vi "sftp.vi"() -> ()   [LabVIEW 2013]
doc: "Illustrate how to read a file using SFTP."
uses:
  libssh2/libssh2_init_default.vi
  libssh2/libssh2_session_handshake_tcp.vi
  libssh2/libssh2.lvlib
panel:
  out "total bytes read":i32
  in  "file":string="/"
  out "file content":string
  out "error out":errorcluster
  in  "password":string
  in  "username":string
  in  "hostname":string
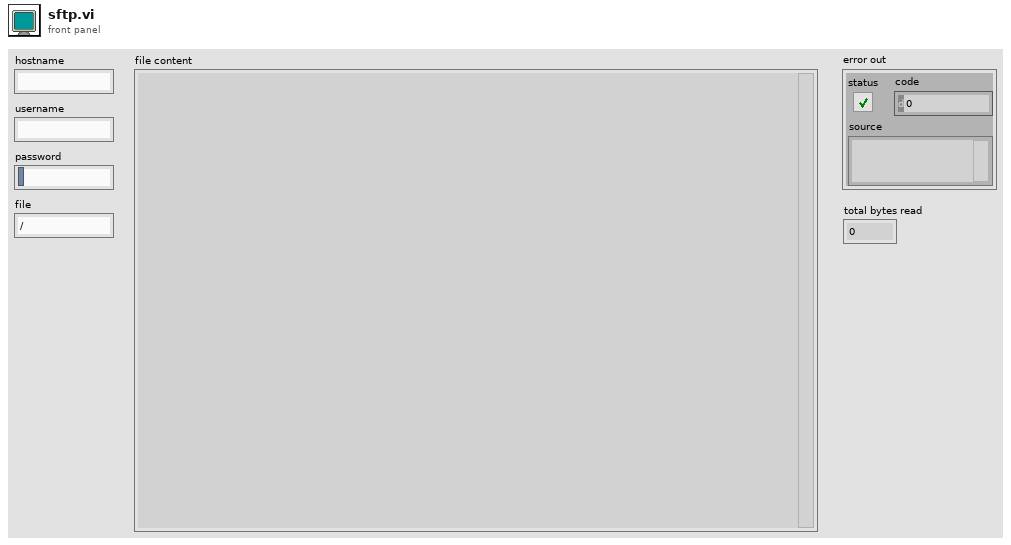
[diagram p1: front panel]
types:
  T1 = typedef "libssh2.lvlib/Session Refnum.ctl" = refnum<k1>
  T2 = typedef "libssh2.lvlib/SFTP Refnum.ctl" = refnum<k1>
  T3 = typedef "libssh2.lvlib/SFTP Handle Refnum.ctl" = refnum<k1>
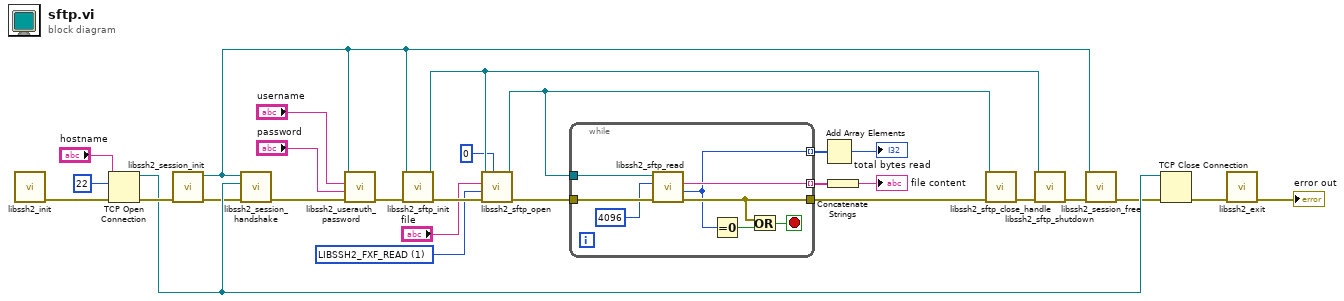
[diagram p0: block diagram]
diagram:
  w5 = u32 1 items=["LIBSSH2_FXF_READ"=1, "LIBSSH2_FXF_WRITE"=2, "LIBSSH2_FXF_APPEND"=4, "LIBSSH2_FXF_CREAT"=8, "LIBSSH2_FXF_TRUNC"=16, "LIBSSH2_FXF_EXCL"=32] ("flags")
  n1 = call-poly "libssh2_init.vi"() -> ("error out"=w27:errorcluster)  [unwired: 11 in]
  n2 = TCP Open Connection(address="hostname", remote port or service name=u16 22, error in (no error)=w27) -> (connection ID=w25:refnum<k5>, error out=w26:errorcluster)  [unwired: 2 in]
  n3 = call "libssh2_session_init.vi"("error in (no error)"=w26) -> ("error out"=w24:errorcluster, "session"=w17:T1)  [unwired: 9 in]
  n4 = call-poly "libssh2_session_handshake.vi"("error in (no error)"=w24, "tcp connection"=w25, "session"=w17) -> ("error out"=w28:errorcluster)  [unwired: 8 in]
  n5 = call "libssh2_userauth_password.vi"("error in (no error)"=w28, "password"="password", "username"="username", "session"=w17) -> ("error out"=w21:errorcluster)  [unwired: 7 in]
  n6 = call "libssh2_sftp_init.vi"("error in (no error)"=w21, "session"=w17) -> ("error out"=w13:errorcluster, "sftp"=w11:T2)  [unwired: 8 in]
  n7 = call "libssh2_sftp_open.vi"("mode"=0, "error in (no error)"=w13, "flags"=w5, "path"="file", "sftp"=w11) -> ("error out"=w12:errorcluster, "sftp handle"=w7:T3)  [unwired: 5 in]
  n8 = while {
    tunnel: w12 -> [w36]
    tunnel: [w33] -> w8
    tunnel: w7 -> [w35]
    tunnel: [w34] -> w4 mode=indexing
    tunnel: [w29] -> w2 mode=indexing
    stop <- w32 stop-if-true
    n9 = call "libssh2_sftp_read.vi"("error in (no error)"=w36, "buffer maxlen"=4096, "sftp handle"=w35) -> ("error out"=w33:errorcluster, "bytes read"=w29:i32, "buffer"=w34:string)  [unwired: 6 in]
    n10 = Equal To 0?(x=w29) -> (x = 0?=w31:bool)
    n11 = Or(x=w33, y=w31) -> (x .or. y?=w32:bool)
  }
  n12 = Add Array Elements(numeric array=w2) -> (sum=→"total bytes read":i32)
  n13 = Concatenate Strings(w4) -> (→"file content":string)
  n14 = call "libssh2_sftp_close_handle.vi"("error in (no error)"=w8, "sftp handle"=w7) -> ("error out"=w9:errorcluster)  [unwired: 9 in]
  n15 = call "libssh2_sftp_shutdown.vi"("error in (no error)"=w9, "sftp"=w11) -> ("error out"=w14:errorcluster)  [unwired: 9 in]
  n16 = call "libssh2_session_free.vi"("error in (no error)"=w14, "session"=w17) -> ("error out"=w16:errorcluster)  [unwired: 9 in]
  n17 = TCP Close Connection(connection ID=w25, error in (no error)=w16) -> (error out=w15:errorcluster)  [unwired: 1 in, 1 out]
  n18 = call "libssh2_exit.vi"("error in (no error)"=w15) -> ("error out"=→"error out":errorcluster)  [unwired: 10 in]
